vi "ERD_Description.vi"(8 "error in":errorcluster, 10 "ERD always show":T1(array[cluster]) {"ERD Number" format="%x"}, 11 "file path":path) -> (0 "error out":errorcluster, 2 "ERD always Out":T1(array[cluster]) {"ERD Number" format="%x"})   [LabVIEW 2021]
uses:
  <vilib>/JDP Science/JSONtext/String Subset.vi
  <vilib>/JDP Science/JSONtext/support/Strip Quotes and Unescape.vi
  <vilib>/JDP Science/JSONtext/support/Unescape JSON string.vi
  <vilib>/JDP Science/JSONtext/Parsing/Parse Full Path or Item Name.vi
  <vilib>/JDP Science/JSONtext/Offset/Find Item Locations by Path.vi
  <vilib>/JDP Science/JSONtext/JSONtext.lvlib
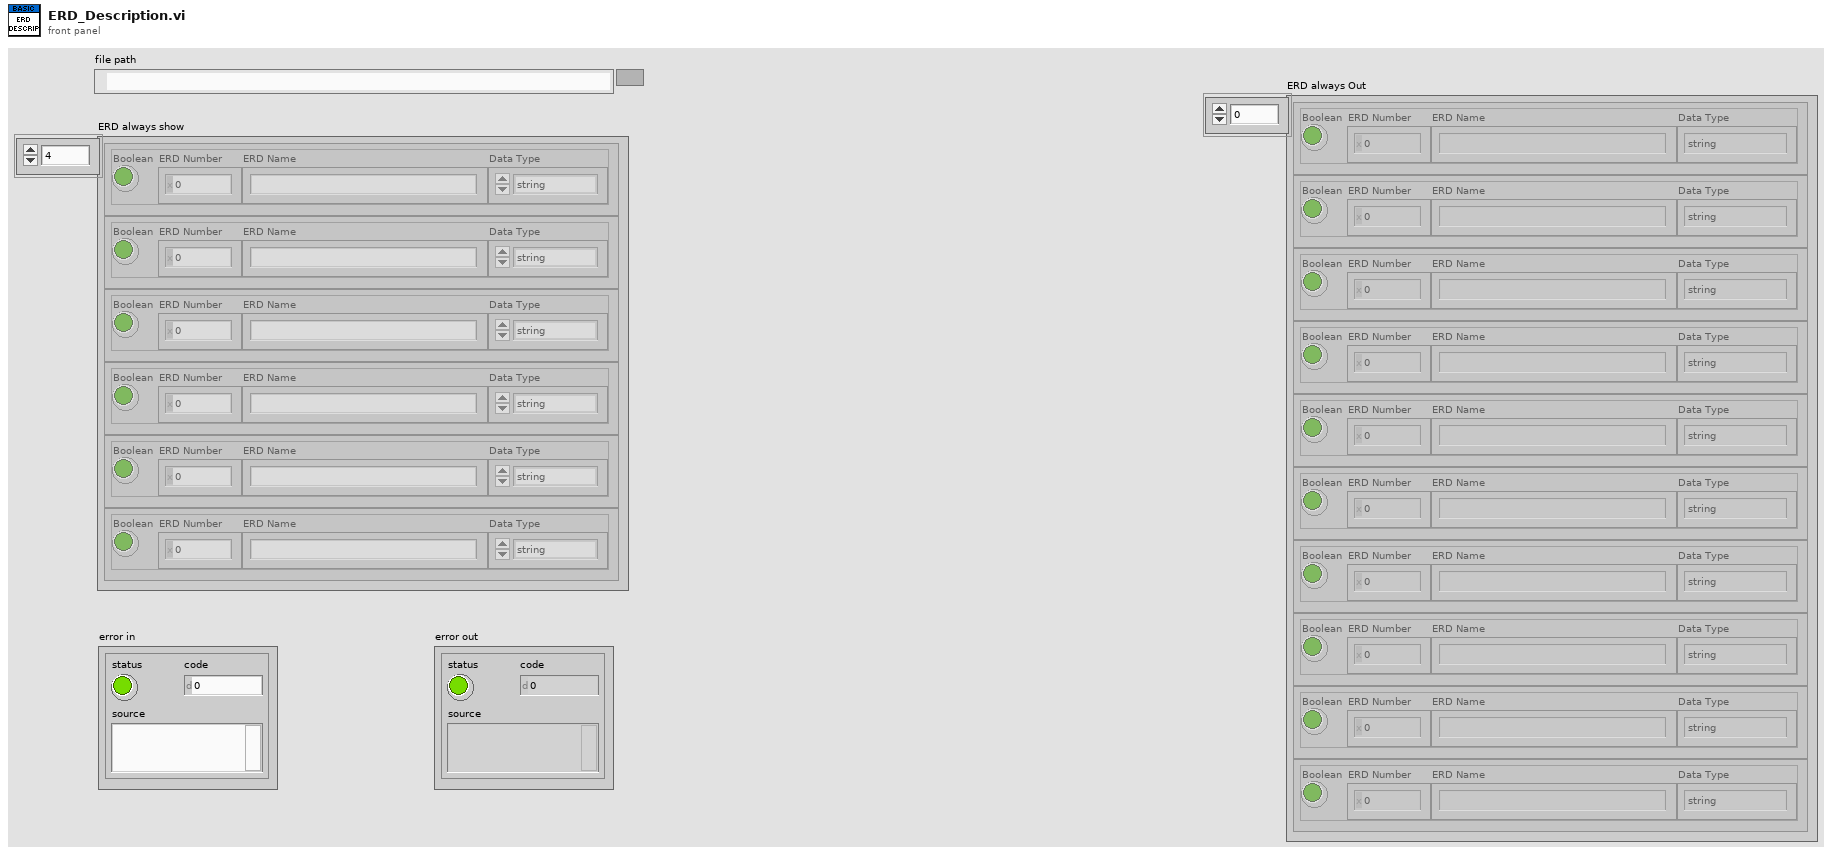
[diagram p1: front panel]
types:
  T1 = cluster{"Boolean":bool, "ERD Number":u16, "ERD Name":string, "Data Type":enum16{"string", "boolean", "uint8_t", "uint16_t", "uint32_t", "uint64_t"}}[]
  T2 = enum16{"open", "replace", "create", "open or create", "replace or create", "replace or create with confirmation"}
  T3 = enum16{"string", "boolean", "uint8_t", "uint16_t", "uint32_t", "uint64_t"}
  T4 = cluster{"Boolean":bool, "ERD Number":u16, "ERD Name":string, "Data Type":enum16{"string", "boolean", "uint8_t", "uint16_t", "uint32_t", "uint64_t"}}
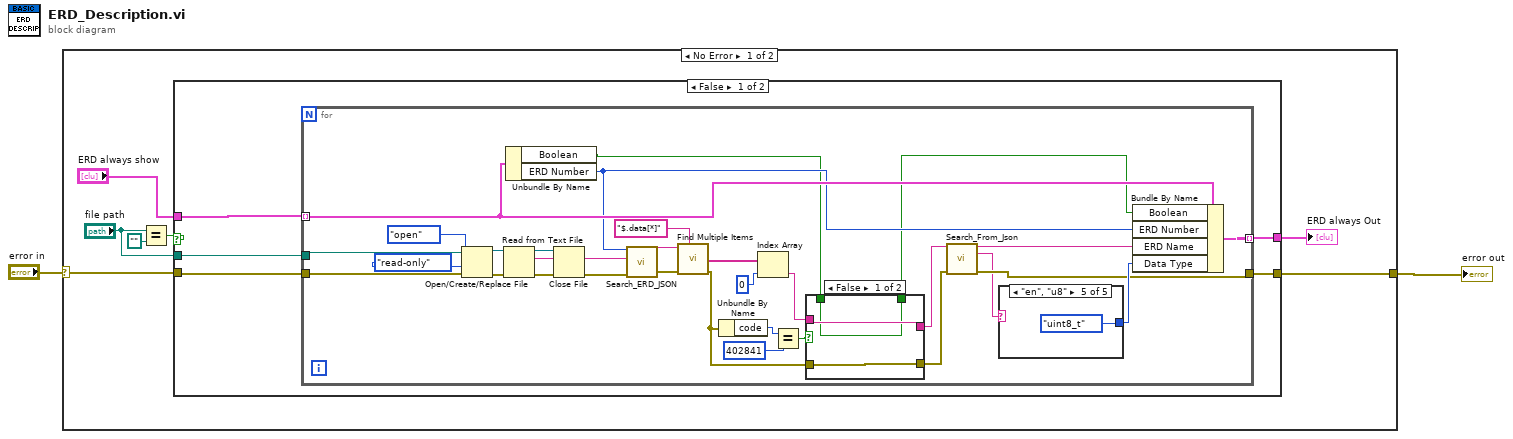
[diagram p0: block diagram]
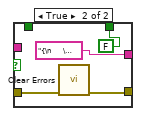
[diagram p2: hidden frame]
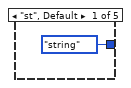
[diagram p3: hidden frame]
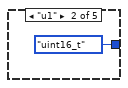
[diagram p4: hidden frame]
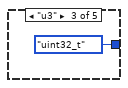
[diagram p5: hidden frame]
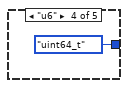
[diagram p6: hidden frame]
diagram:
  n1 = case shown="No Error" "error in" {
    selector: "error in" -> [w9 w60]
    tunnel: [w8 w60] -> w1
    frame No Error {
      n2 = Equal?(x="file path", y=path "") -> (x = y?=w6:bool)
      n3 = case shown="False" w6 {
        tunnel: w9 -> [w14 w59]
        tunnel: [w13 w59] -> w8
        tunnel: "ERD always show" -> [w10 w58]
        tunnel: [w12 w58] -> w4
        tunnel: "file path" -> [w11 _]
        frame False {
          n4 = for {
            tunnel: w10 -> [w34] mode=indexing
            tunnel: w14 -> [w38]
            tunnel: [w25] -> w13
            tunnel: w11 -> [w39]
            tunnel: [w32] -> w12 mode=indexing
            n5 = Open/Create/Replace File(file path (use dialog)=w39, error in=w38, operation (0:open)=T2."open", access (0:read/write)=enum16{"read/write", "read-only", "write-only"}."read-only") -> (refnum out=w44:refnum<file>, error out=w42:errorcluster)  [unwired: 2 in, 1 out]
            n6 = Read from Text File(file (use dialog)=w44, error in=w42) -> (refnum out=w45:refnum<file>, text=w37:string, error out=w43:errorcluster)  [unwired: 2 in, 1 out]
            n7 = Unbundle By Name(w34) -> ("Boolean"=w16:bool, "ERD Number"=w33:u16)
            n8 = Close File(refnum=w45, error in=w43) -> (error out=w27:errorcluster)  [unwired: 1 out]
            n9 = call "Search_ERD_JSON.vi"("ERD Number"=w33, "JSON Text"=w37, "error in"=w27) -> ("ERD"=w35:string, "error out"=w26:errorcluster)  [unwired: 11 in]
            n10 = call <vilib>:"Find Multiple Items.vi"("$Path or Item Name"="$.data[*]", "error in (no error)"=w26, "JSON"=w35) -> ("error out"=w21:errorcluster, "<JSON>"=w28:string[])  [unwired: 5 in, 2 out]
            n11 = Unbundle By Name(w21) -> ("code"=w24:i32)
            n12 = Index Array(array=w28, index=0) -> (element=w18:string)
            n13 = Equal?(x=w24, y=402841) -> (x = y?=w22:bool)
            n14 = case shown="False" w22 {
              tunnel: w21 -> [w48 w52]
              tunnel: [w48 w51] -> w20
              tunnel: [w47 "{\n      \"name\": \"No found\",\n      \"type\": \"string\",\n      \"offset\": 0,\n      \"size\": 0\n    }" ("element")] -> w19
              tunnel: w18 -> [w47 _]
              tunnel: [w46 FALSE] -> w17
              tunnel: w16 -> [w46 _]
              frame False {
              }
              frame True {
                n15 = call <vilib>:"Clear Errors.vi"("error in (no error)"=w52) -> ("error out"=w51:errorcluster)  [unwired: 5 in, 1 out]
              }
            }
            n16 = call "Search_From_Json.vi"("Data JSON"=w19, "error in"=w20) -> ("Name"=w30:string, "Type"=w15:string, "error IO"=w25:errorcluster)  [unwired: 9 in, 2 out]
            n17 = case shown="\"en\", \"u8\"" w15 {
              tunnel: [T3."string" ("Data Type") T3."uint16_t" ("Data Type") T3."uint32_t" ("Data Type") T3."uint64_t" ("Data Type") T3."uint8_t" ("Data Type")] -> w29
              frame "st", Default {
              }
              frame "u1" {
              }
              frame "u3" {
              }
              frame "u6" {
              }
              frame "en", "u8" {
              }
            }
            n18 = Bundle By Name(cluster=w34, "Boolean"=w17, "ERD Number"=w33, "ERD Name"=w30, "Data Type"=w29) -> (w32:T4)
          }
        }
        frame True {
        }
      }
      "ERD always Out" <- w4
    }
    frame Error {
    }
  }
  "error out" <- w1
